vi "Bool Ctl False.vi"(0 "Control Ref":refnum<vi>) -> ()   [LabVIEW 2015]
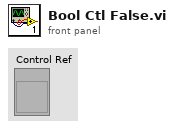
[diagram p1: front panel]
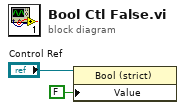
[diagram p0: block diagram]
diagram:
  n1 = property class="Bool (strict)"(reference="Control Ref", "Value"=FALSE) -> ()  [unwired: 1 in, 2 out]
